vi "PNS Variabler Taktmerker III.vi"(8 "error in (no error)":errorcluster caption="Fehler (Eingang, kein Fehler)", 9 "Aus in sec.":dbl, 10 "Ein in sec.":dbl, 11 "Aktion":T1) -> (0 "error out":errorcluster caption="Fehler (Ausgang)", 2 "Takt":bool, 3 "Aktion":T1)   [LabVIEW 2020, in "PNS.lvlib"]
doc: "Von cRIO kopiert - Takten in \"lesen\" gepflanzt, sonst loop das immer nur ohne takten,\nund zusätzlich bei III statt zählen einen Zeitstempel,\nweil \"lesen\" im FGV Modbus KommunikationOO vi öfter aufgerufen wird, und dann jedesmal hochgezählt wird !\n\nriw - 30.08.2019"
uses:
  PNS.lvlib
  Aktion PNS FGV variabler Taktmerker.ctl
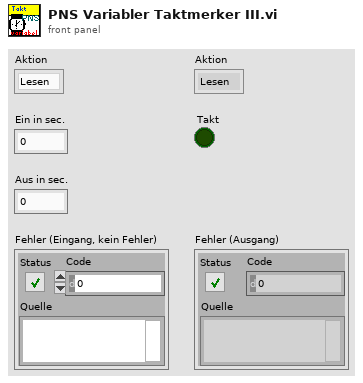
[diagram p1: front panel]
types:
  T1 = typedef "PNS.lvlib/Aktion PNS FGV variabler Taktmerker.ctl" = enum16{"Lesen", "aktiv", "inaktiv", "Werte schreiben"}
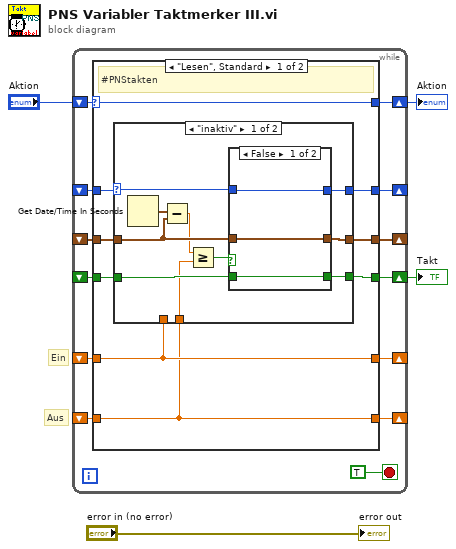
[diagram p0: block diagram]
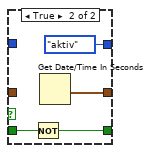
[diagram p2: hidden frame]
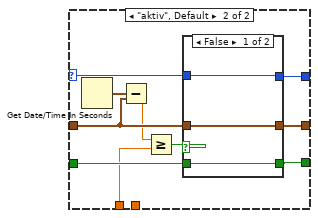
[diagram p3: hidden frame]
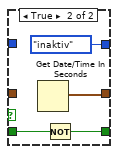
[diagram p4: hidden frame]
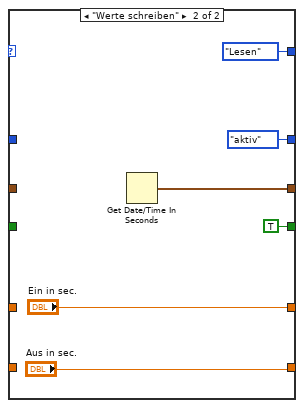
[diagram p5: hidden frame]
diagram:
  # "Aus"
  # "Ein"
  n1 = while {
    shift-right: [w15] -> _
    shift-left: _ -> [w14]
    shift-right: [w13] -> w2
    shift-left: _ -> [w12]
    shift-right: [w11] -> w3
    shift-left: "Aktion" -> [w16]
    shift-right: [w10] -> _
    shift-left: _ -> [w7]
    shift-right: [w9] -> _
    shift-left: _ -> [w8]
    shift-right: [w6] -> _
    shift-left: _ -> [w5]
    stop <- TRUE stop-if-true
    n2 = case shown="\"Lesen\", Standard" w16 {
      selector: w16 -> [w26 _]
      tunnel: [w21 w64] -> w15
      tunnel: w14 -> [w22 _]
      tunnel: [w23 TRUE] -> w13
      tunnel: w12 -> [w24 _]
      tunnel: [w26 Aktion_PNS_FGV_variabler_Taktmerker."Lesen" ("Aktion")] -> w11
      tunnel: [w25 "Ein in sec."] -> w10
      tunnel: [w20 "Aus in sec."] -> w9
      tunnel: w8 -> [w20 _]
      tunnel: w7 -> [w25 _]
      tunnel: w5 -> [w19 _]
      tunnel: [w18 Aktion_PNS_FGV_variabler_Taktmerker."aktiv" ("Aktion")] -> w6
      frame "Lesen", Default {
        # "#PNStakten"
        n3 = case shown="\"inaktiv\"" w19 {
          selector: w19 -> [w32 w49]
          tunnel: w25 -> [_ w45]
          tunnel: w24 -> [w33 w53]
          tunnel: [w34 w52] -> w23
          tunnel: w22 -> [w30 w47]
          tunnel: [w35 w50] -> w21
          tunnel: w20 -> [w28 _]
          tunnel: [w27 w44] -> w18
          frame "inaktiv" {
            n4 = Get Date/Time In Seconds() -> (seconds since 1Jan1904=w31:timestamp)
            n5 = Subtract(x=w31, y=w30) -> (x-y=w29:dbl)
            n6 = Greater Or Equal?(x=w29, y=w28) -> (x >= y?=w36:bool)
            n7 = case shown="False" w36 {
              tunnel: [w39 w41] -> w35
              tunnel: w30 -> [w39 _]
              tunnel: [w38 w43] -> w34
              tunnel: w33 -> [w38 w42]
              tunnel: w32 -> [w37 _]
              tunnel: [w37 Aktion_PNS_FGV_variabler_Taktmerker."aktiv" ("Aktion")] -> w27
              frame False {
              }
              frame True {
                n8 = Not(x=w42) -> (.not. x?=w43:bool)
                n9 = Get Date/Time In Seconds() -> (seconds since 1Jan1904=w41:timestamp)
              }
            }
          }
          frame "aktiv", Default {
            n10 = Get Date/Time In Seconds() -> (seconds since 1Jan1904=w48:timestamp)
            n11 = Subtract(x=w48, y=w47) -> (x-y=w46:dbl)
            n12 = Greater Or Equal?(x=w46, y=w45) -> (x >= y?=w51:bool)
            n13 = case shown="False" w51 {
              tunnel: [w56 w58] -> w50
              tunnel: w47 -> [w56 _]
              tunnel: [w55 w60] -> w52
              tunnel: w53 -> [w55 w59]
              tunnel: w49 -> [w54 _]
              tunnel: [w54 Aktion_PNS_FGV_variabler_Taktmerker."inaktiv" ("Aktion")] -> w44
              frame False {
              }
              frame True {
                n14 = Get Date/Time In Seconds() -> (seconds since 1Jan1904=w58:timestamp)
                n15 = Not(x=w59) -> (.not. x?=w60:bool)
              }
            }
          }
        }
      }
      frame "Werte schreiben" {
        n16 = Get Date/Time In Seconds() -> (seconds since 1Jan1904=w64:timestamp)
      }
    }
  }
  "Aktion" <- w3
  "Takt" <- w2
  "error out" <- "error in (no error)"
